vi "AI Read.vi"(7 "AI line":T1=4000 items=["ModA/AI0"=4000, "ModA/AI1"=4001, "ModA/AI2"=4002, "ModA/AI3"=4003, "ModA/AI4"=4004, "ModA/AI5"=4005, "ModA/AI6"=4006, "ModA/AI7"=4007, "ModA/AI8"=4008, "ModA/AI9"=4009], 8 "error in (no error)":errorcluster, 11 "direct IO in":refnum<class "NI_Robotics_Starter Kit Direct IO_FPGA.lvclass">) -> (0 "error out":errorcluster, 2 "data":dbl, 3 "direct IO out":refnum<class "NI_Robotics_Starter Kit Direct IO_FPGA.lvclass">)   [LabVIEW 2017, in "NI_Robotics_Starter Kit Direct IO_FPGA.lvclass"]
uses:
  <vilib>/robotics/Starter Kit/FPGA Direct IO/NI_Robotics_Starter Kit Direct IO_FPGA.lvclass
  <vilib>/robotics/Starter Kit/Direct IO/AI Lines.ctl
  <vilib>/robotics/Starter Kit/FPGA Direct IO/NI_Robotics_Starter Kit Direct IO_FPGA.lvclass/NI_Robotics_Starter Kit Direct IO_FPGA.ctl
  <vilib>/rvi/errors/niLvFpgaAdjustHostInterfaceError.vi
  <vilib>/Utility/error.llb/Error Cluster From Error Code.vi
  <vilib>/robotics/Starter Kit/FPGA Direct IO/Direct IO FPGA Ref.ctl
  <vilib>/rvi/interface/nirviReadWriteControl/nirviReadWriteControl.xnode
  NiFpgaLv.dll
  <vilib>/rvi/interface/Simulation/niFpgaSimulationCallBeginRW.vi
  <vilib>/robotics/Starter Kit/Direct IO/NI_Robotics_Starter Kit Direct IO.lvclass
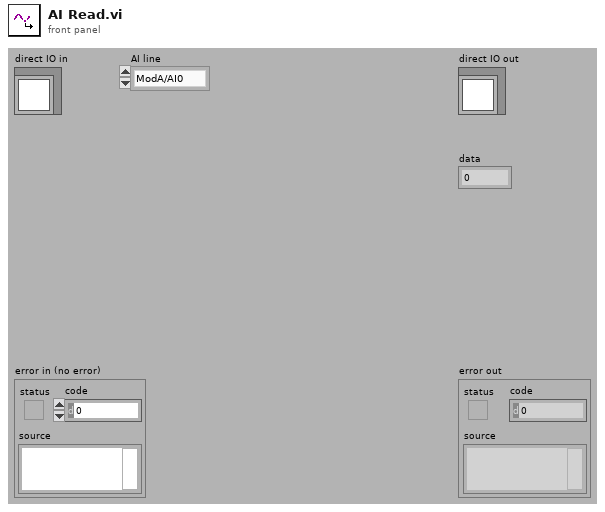
[diagram p1: front panel]
types:
  T1 = typedef "NI_Robotics_Starter Kit Direct IO.lvclass/AI Lines.ctl" = u16
  T2 = typedef "NI_Robotics_Starter Kit Direct IO_FPGA.lvclass/Direct IO FPGA Ref.ctl" = refnum<k20>
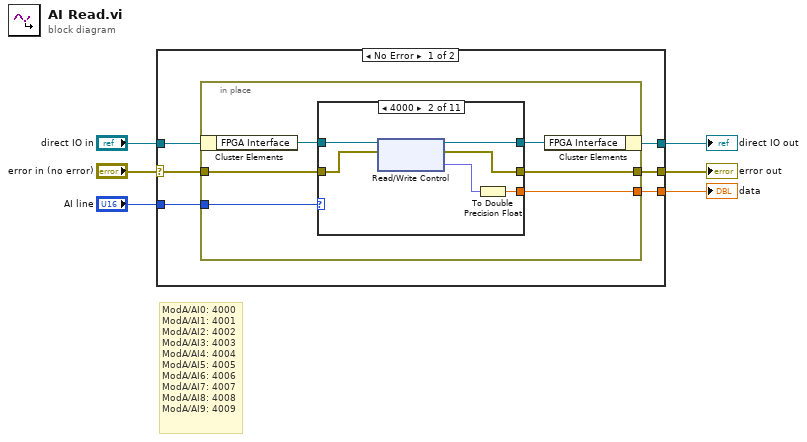
[diagram p0: block diagram]
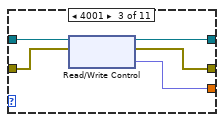
[diagram p3: hidden frame]
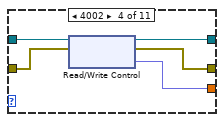
[diagram p4: hidden frame]
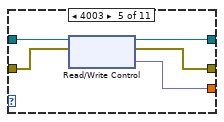
[diagram p5: hidden frame]
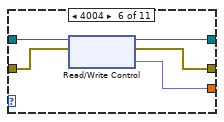
[diagram p6: hidden frame]
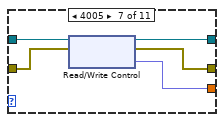
[diagram p7: hidden frame]
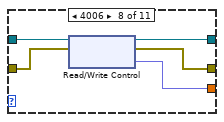
[diagram p8: hidden frame]
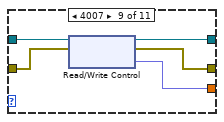
[diagram p9: hidden frame]
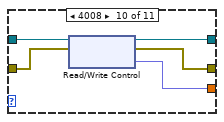
[diagram p10: hidden frame]
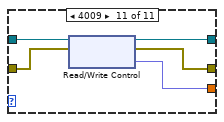
[diagram p11: hidden frame]
diagram:
  # "ModA/AI0: 4000\nModA/AI1: 4001\nModA/AI2: 4002\nModA/AI3: 4003\nModA/AI4: 4004\nModA/AI5: 4005\nModA/AI6: 4006\nModA/AI7: 4007\nModA/AI8: 4008\nModA/AI9: 4009"
  n1 = case shown="No Error" "error in (no error)" {
    selector: "error in (no error)" -> [w10 w73]
    tunnel: [w9 w73] -> w3
    tunnel: "direct IO in" -> [w12 w72]
    tunnel: [w8 w72] -> w2
    tunnel: "AI line" -> [w11 _]
    tunnel: [w7 _] -> w1
    frame No Error {
      n2 = in-place {
        in-place-border: w11 -> [w18]
        in-place-border: w10 -> [w16]
        in-place-border: [w14] -> w9
        in-place-border: [w13] -> w7
        n3 = in-place-cluster #1(w12) -> ("FPGA Interface"=w17:T2)
        n4 = case shown="4000" w18 {
          tunnel: w17 -> [w20 w26 w31 w36 w41 w46 w51 w56 w61 w66 w71]
          tunnel: w16 -> [w19 w25 w30 w35 w40 w45 w50 w55 w60 w65 w70]
          tunnel: [w20 w24 w29 w34 w39 w44 w49 w54 w59 w64 w69] -> w15
          tunnel: [w19 w23 w28 w33 w38 w43 w48 w53 w58 w63 w68] -> w14
          tunnel: [_ w21 w27 w32 w37 w42 w47 w52 w57 w62 w67] -> w13
          frame Default {
          }
          frame 4000 {
            n5 = xnode "Read/Write Control"("FPGA VI Reference In"=w26, "error in"=w25) -> ("FPGA VI Reference Out"=w24:T2, "error out"=w23:errorcluster, "ModA/AI0"=w22:fxp<+/-,26,5>)
            n6 = To Double Precision Float(number=w22) -> (double precision float=w21:dbl)
          }
          frame 4001 {
            n7 = xnode "Read/Write Control"("FPGA VI Reference In"=w31, "error in"=w30) -> ("FPGA VI Reference Out"=w29:T2, "error out"=w28:errorcluster, "ModA/AI1"=w27:fxp<+/-,26,5>)
          }
          frame 4002 {
            n8 = xnode "Read/Write Control"("FPGA VI Reference In"=w36, "error in"=w35) -> ("FPGA VI Reference Out"=w34:T2, "error out"=w33:errorcluster, "ModA/AI2"=w32:fxp<+/-,26,5>)
          }
          frame 4003 {
            n9 = xnode "Read/Write Control"("FPGA VI Reference In"=w41, "error in"=w40) -> ("FPGA VI Reference Out"=w39:T2, "error out"=w38:errorcluster, "ModA/AI3"=w37:fxp<+/-,26,5>)
          }
          frame 4004 {
            n10 = xnode "Read/Write Control"("FPGA VI Reference In"=w46, "error in"=w45) -> ("FPGA VI Reference Out"=w44:T2, "error out"=w43:errorcluster, "ModA/AI4"=w42:fxp<+/-,26,5>)
          }
          frame 4005 {
            n11 = xnode "Read/Write Control"("FPGA VI Reference In"=w51, "error in"=w50) -> ("FPGA VI Reference Out"=w49:T2, "error out"=w48:errorcluster, "ModA/AI5"=w47:fxp<+/-,26,5>)
          }
          frame 4006 {
            n12 = xnode "Read/Write Control"("FPGA VI Reference In"=w56, "error in"=w55) -> ("FPGA VI Reference Out"=w54:T2, "error out"=w53:errorcluster, "ModA/AI6"=w52:fxp<+/-,26,5>)
          }
          frame 4007 {
            n13 = xnode "Read/Write Control"("FPGA VI Reference In"=w61, "error in"=w60) -> ("FPGA VI Reference Out"=w59:T2, "error out"=w58:errorcluster, "ModA/AI7"=w57:fxp<+/-,26,5>)
          }
          frame 4008 {
            n14 = xnode "Read/Write Control"("FPGA VI Reference In"=w66, "error in"=w65) -> ("FPGA VI Reference Out"=w64:T2, "error out"=w63:errorcluster, "ModA/AI8"=w62:fxp<+/-,26,5>)
          }
          frame 4009 {
            n15 = xnode "Read/Write Control"("FPGA VI Reference In"=w71, "error in"=w70) -> ("FPGA VI Reference Out"=w69:T2, "error out"=w68:errorcluster, "ModA/AI9"=w67:fxp<+/-,26,5>)
          }
        }
        n16 = in-place-cluster #1("FPGA Interface"=w15) -> (w8:refnum<class "NI_Robotics_Starter Kit Direct IO_FPGA.lvclass">)
      }
    }
    frame Error {
    }
  }
  "error out" <- w3
  "direct IO out" <- w2
  "data" <- w1
